vi "Condition Private Data.vi"(8 "error in":errorcluster, 9 "Ref.Private Data Cluster":refnum<vi>, 10 "Ref.Private Data Control":refnum<vi>) -> (0 "error out":errorcluster)   [LabVIEW 2025, in "_Msg Rescript.lvlib" / "_Msg Rescript.lvclass"]
uses:
  _Msg Rescript.lvclass
  _Msg Rescript.lvclass/_Msg Rescript.ctl
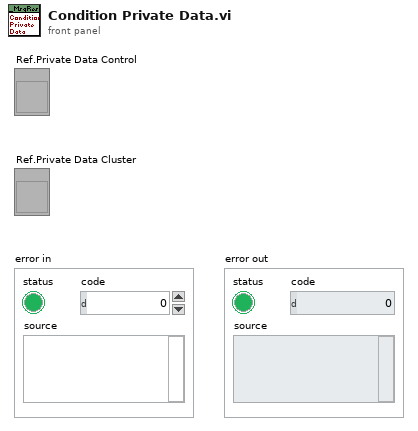
[diagram p1: front panel]
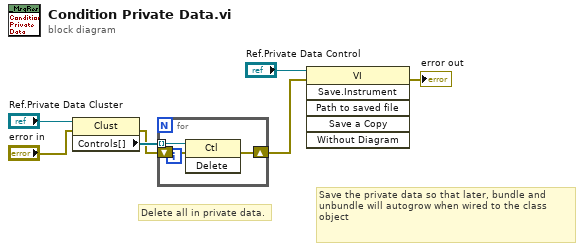
[diagram p0: block diagram]
diagram:
  # "Delete all in private data."
  # "Save the private data so that later, bundle and unbundle will autogrow when wired to the class object"
  n1 = property class="Clust"(reference="Ref.Private Data Cluster", error in="error in") -> (error out=w6:errorcluster, "Controls[]"=w7:refnum<vi>[])  [unwired: 1 out]
  n2 = for {
    tunnel: w7 -> [w10] mode=indexing
    shift-right: [w8] -> w5
    shift-left: w6 -> [w9]
    n3 = invoke class="Ctl" method="Delete"(reference=w10, error in=w9) -> (error out=w8:errorcluster)  [unwired: 1 in, 2 out]
  }
  n4 = invoke class="VI" method="Save.Instrument"(reference="Ref.Private Data Control", error in=w5) -> (error out=→"error out":errorcluster)  [unwired: 4 in, 5 out]
